vi "rs3 delete context.vi"(8 "error in (no error)":errorcluster, 11 "context":u64) -> (0 "error out":errorcluster)   [LabVIEW 2023]
doc: "The final command should be to delete the CONTEXT, after all sensors, and devices have been stopped and deleted."
panel:
  # "RS3 Delete Context"
  # "(C) Intel Corp. 2017,  AGJ"
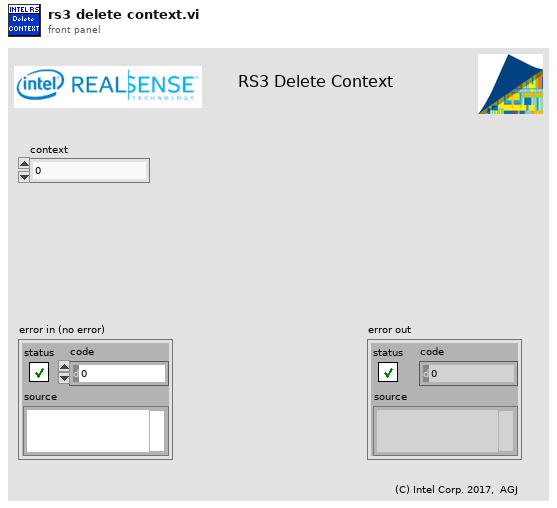
[diagram p1: front panel]
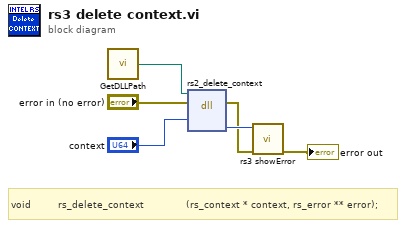
[diagram p0: block diagram]
diagram:
  # "void         rs_delete_context              (rs_context * context, rs_error ** error);"
  n1 = call "GetDLLPath.vi"() -> ("DLL Path"=w1:path)
  n2 = dll-call lib="C:/STEAMSyndicate/RealSenseWrappers/VI Wrappers (add ons) Public/RealSense/realsense2.dll" fn="rs2_delete_context"(path in=w1, error in="error in (no error)", "context"="context") -> (error out=w3:errorcluster, "error"=w4:u64)  [unwired: 4 in, 1 out]
  n3 = call "rs3 showError.vi"("error in (no error)"=w3, "error"=w4) -> ("error out"=→"error out":errorcluster)  [unwired: 5 in, 4 out]
